vi "Exceptions.vi"() -> ()   [LabVIEW 2020, in "Silly Billy.lvlib"]
uses:
  Silly Billy.lvlib
panel:
  in  "Exceptions":map{string[], string[]}(c390)={["column"]=["col", "umn"], ["columns"]=["col", "umns"], ["at", "tribute"]=["at", "trib", "ute"], ["at", "tributes"]=["at", "trib", "utes"]}
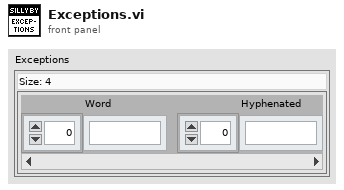
[diagram p1: front panel]
diagram:
